vi "Write all custom data.vi"(8 "error in (no error)":errorcluster, 9 "Custom Data":string[](array[string]), 10 "Keys":string[](array[string]), 11 "img":T1) -> (0 "error out":errorcluster, 3 "Image (duplicate)":T1)   [LabVIEW 2013]
doc: "This .vi write a series of custom data to the image buff."
uses:
  <vilib>/vision/Image Controls.llb/IMAQ Image.ctl
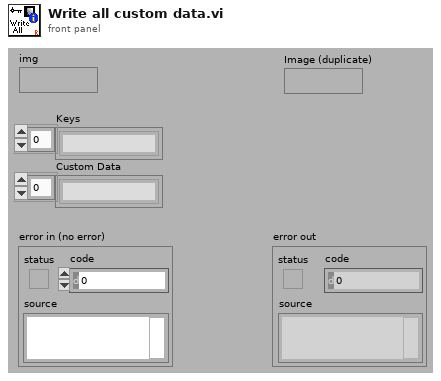
[diagram p1: front panel]
types:
  T1 = typedef "IMAQ Image.ctl" = refnum<image>
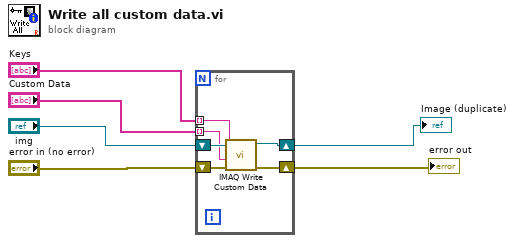
[diagram p0: block diagram]
diagram:
  n1 = for {
    shift-right: [w11] -> w4
    shift-left: "img" -> [w12]
    tunnel: "Keys" -> [w10] mode=indexing
    shift-right: [w8] -> w5
    shift-left: "error in (no error)" -> [w9]
    tunnel: "Custom Data" -> [w7] mode=indexing
    n2 = call "IMAQ Write Custom Data"("error in (no error)"=w9, "Custom Data In"=w7, "Key"=w10, "Image"=w12) -> ("error out"=w8:errorcluster, "Image Out"=w11:T1)  [unwired: 6 out]
  }
  "error out" <- w5
  "Image (duplicate)" <- w4
